vi "FT_Set_Characters.vi"(1 "Characters":T1 {"Error Character" format="%x"; "Event Character" format="%x"}, 2 "Handle":u32) -> (0 "FT_Status":u32(ring) items=["FT_OK", "FT_INVALID_HANDLE", "FT_DEVICE_NOT_FOUND", "FT_DEVICE_NOT_OPENED", "FT_IO_ERROR", "FT_INSUFFICIENT_RESOURCES", "FT_INVALID_PARAMETER", "FT_INVALID_BAUD_RATE", "FT_DEVICE_NOT_OPENED_FOR_ERASE", "FT_DEVICE_NOT_OPENED_FOR_WRITE", "FT_FAILED_TO_WRITE_DEVICE", "FT_EEPROM_READ_FAILED", "FT_EEPROM_WRITE_FAILED", "FT_EEPROM_ERASE_FAILED", "FT_EEPROM_NOT_PRESENT", "FT_EEPROM_NOT_PROGRAMMED", "FT_INVALID_ARGS", "FT_NOT_SUPPORTED", "FT_OTHER_ERROR"])   [LabVIEW 2019, in "D2XX_Functions.lvlib"]
uses:
  D2XX_Functions.lvlib
  CDM v2.12.36.4 WHQL Certified/i386/ftd2xx.dll
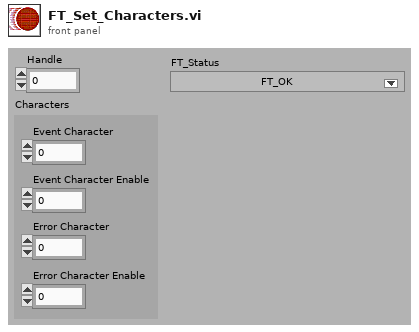
[diagram p1: front panel]
types:
  T1 = cluster{"Event Character":u8, "Event Character Enable":u8, "Error Character":u8, "Error Character Enable":u8}
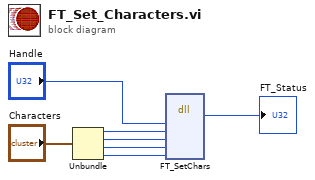
[diagram p0: block diagram]
diagram:
  n1 = Unbundle("Characters") -> ("Event Character"=w4:u8, "Event Character Enable"=w3:u8, "Error Character"=w2:u8, "Error Character Enable"=w1:u8)
  n2 = dll-call lib="C:/Users/patrick/Documents/GitHub/Relay-Box/lvsrc/CDM v2.12.36.4 WHQL Certified/i386/FTD2XX.dll" fn="FT_SetChars"("Handle"="Handle", "EventCharacter"=w4, "EventCharacterEnable"=w3, "ErrorCharacter"=w2, "ErrorCharacterEnable"=w1) -> ("FT_Status"=→"FT_Status":u32)  [unwired: 8 in, 2 out]
